vi "State_Machine.vi"(8 "error in (no error)":errorcluster caption="entrée d'erreur (pas d'erreur)", 11 "Wait_CloseFixture en entrée":refnum<class "Operator_Control.lvclass">) -> (0 "error out":errorcluster caption="sortie d'erreur", 2 "Json_String":string, 3 "Wait_CloseFixture en sortie":refnum<class "Operator_Control.lvclass">)   [LabVIEW 2020, in "Library Test.lvlib" / "Operator_Control.lvclass"]
uses:
  Operator_Control.lvclass
  C:/Users/ngarcin/OneDrive - Altyor/Standard TB/Class/Test/Test (Default)/Test (Default).lvclass
  Popup/Class Popup Operator_Validation/Class Popup Operator_Validation/Class Popup Operator_Validation.lvclass
  C:/Users/ngarcin/OneDrive - Altyor/Standard TB/Class/Popup/Class Popup Operator_Validation/Class Popup Operator_Validation (Default)/Class Popup Operator_Validation (Virtual).lvclass
  C:/Users/ngarcin/OneDrive - Altyor/Standard TB/Class/Popup/Class Popup (Main)/Class Popup (Main).lvclass
  Operator_Control.lvclass/Operator_Control.ctl
  Commun VI/Library Commun.lvlib
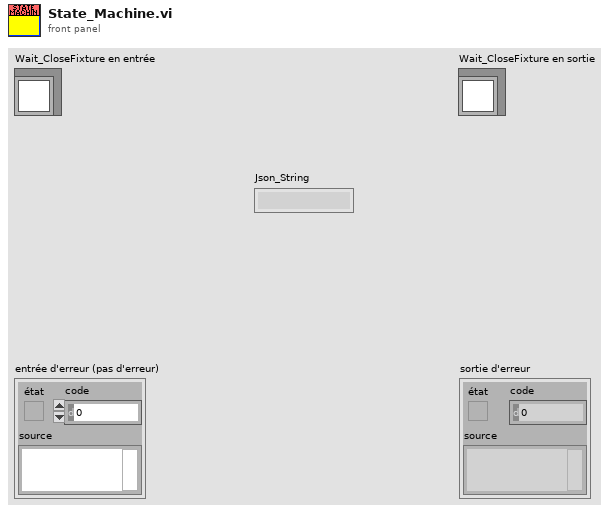
[diagram p1: front panel]
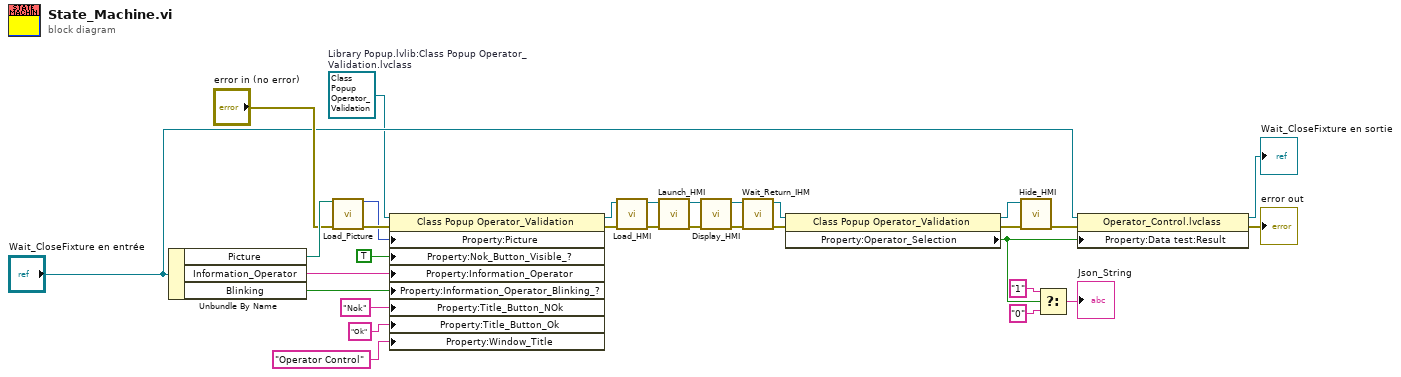
[diagram p0: block diagram]
diagram:
  w2 = refnum<class "Class Popup Operator_Validation.lvclass"> refnum  # Library Popup.lvlib:Class Popup Operator_Validation.lvclass
  n1 = Unbundle By Name("Wait_CloseFixture en entrée") -> ("Picture"=w24:path, "Information_Operator"=w27:string, "Blinking"=w26:bool)
  n2 = call "Load_Picture.vi"("Chemin In"=w24, "error in (no error)"="error in (no error)") -> ("Img Out"=w23:picture, "error out"=w25:errorcluster)  [unwired: 11 in, 1 out]
  n3 = property class="Class Popup Operator_Validation"(reference=w2, error in=w25, "Property:Picture"=w23, "Property:Nok_Button_Visible_?"=TRUE ("Nok_Button_Visible_?"), "Property:Information_Operator"=w27, "Property:Information_Operator_Blinking_?"=w26, "Property:Title_Button_NOk"="Nok" ("Title_Button_NOk"), "Property:Title_Button_Ok"="Ok" ("Title_Button_Ok"), "Property:Window_Title"="Operator Control" ("Window_Title")) -> (reference out=w30:refnum<class "Class Popup Operator_Validation.lvclass">, error out=w29:errorcluster)
  n4 = call-dynamic "Load_HMI.vi"("error in (no error)"=w29, "Class Popup (Default) en entrée"=w30) -> ("error out"=w20:errorcluster, "Class Popup (Default) en sortie"=w21:refnum<class "Class Popup Operator_Validation.lvclass">)  [unwired: 8 in]
  n5 = call-dynamic "Launch_HMI.vi"("error in (no error)"=w20, "Class Popup (Default) en entrée"=w21) -> ("error out"=w31:errorcluster, "Class Popup (Default) en sortie"=w22:refnum<class "Class Popup Operator_Validation.lvclass">)  [unwired: 8 in]
  n6 = call-dynamic "Display_HMI.vi"("error in (no error)"=w31, "Class Popup (Default) en entrée"=w22) -> ("error out"=w19:errorcluster, "Class Popup (Default) en sortie"=w18:refnum<class "Class Popup Operator_Validation.lvclass">)  [unwired: 8 in]
  n7 = call-dynamic "Wait_Return_IHM.vi"("error in (no error)"=w19, "Class Popup (Default) en entrée"=w18) -> ("error out"=w14:errorcluster, "Class Popup (Default) en sortie"=w16:refnum<class "Class Popup Operator_Validation.lvclass">)  [unwired: 8 in]
  n8 = property class="Class Popup Operator_Validation"(reference=w16, error in=w14) -> (reference out=w15:refnum<class "Class Popup Operator_Validation.lvclass">, error out=w13:errorcluster, "Property:Operator_Selection"=w8:bool)
  n9 = call-dynamic "Hide_HMI.vi"("error in (no error)"=w13, "Class Popup (Default) en entrée"=w15) -> ("error out"=w12:errorcluster)  [unwired: 8 in, 1 out]
  n10 = Select(t="1", s=w8, f="0") -> (s? t:f=→"Json_String":string)
  n11 = property class="Operator_Control.lvclass"(reference="Wait_CloseFixture en entrée", error in=w12, "Property:Data test:Result"=w8) -> (reference out=→"Wait_CloseFixture en sortie":refnum<class "Operator_Control.lvclass">, error out=→"error out":errorcluster)
